vi "cDAQ Abort Digitize.vi"(8 "error in":errorcluster, 11 "cdaq session in":T1={"mclk [Hz]"=12800000.0, "ADC task"="", "mclk reference"="", "fs [Hz]"=50000.0, "queue adc cmd"=refnum, "queue adc data"=refnum, "adc proc ref"=refnum, "channels"=[], "last channels"=[], "timeout"=timestamp(0 s since 1904-01-01), "N"=1000, "mclk mode"=enum."Free running", "ext mclk source"=""} {"last channels"."Channel id" min=0 step=1; "channels"."Channel id" min=0 step=1}) -> (0 "error out":errorcluster, 3 "cdaq session out":T1={"mclk [Hz]"=12800000.0, "ADC task"="", "mclk reference"="", "fs [Hz]"=50000.0, "queue adc cmd"=refnum, "queue adc data"=refnum, "adc proc ref"=refnum, "channels"=[], "last channels"=[], "timeout"=timestamp(0 s since 1904-01-01), "N"=1000, "mclk mode"=enum."Free running", "ext mclk source"=""} {"last channels"."Channel id" min=0 step=1; "channels"."Channel id" min=0 step=1})   [LabVIEW 2020]
uses:
  cDAQ Session.ctl
  low_level_old/cdaq_anal_adc_command.ctl
  low_level_old/cdaq_anal_adc_data.ctl
  cDAQ Virtual Channel.ctl
  cDAQ Master Clock Mode.ctl
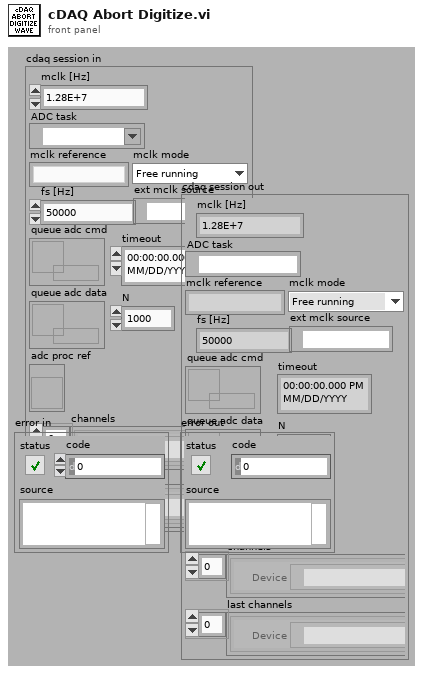
[diagram p1: front panel]
types:
  T1 = typedef "cDAQ Session.ctl" = cluster{"mclk [Hz]":dbl, "ADC task":refnum<k21>, "mclk reference":string, "fs [Hz]":dbl, "queue adc cmd":refnum<queue>, "queue adc data":refnum<queue>, "adc proc ref":refnum<vi>, "channels":T2[], "last channels":T2[], "timeout":timestamp, "N":i32, "mclk mode":T3, "ext mclk source":tag}
  T2 = typedef "cDAQ Virtual Channel.ctl" = cluster{"Device":tag, "Channel id":i32, "btn clr":bool, "btn up":bool, "btn down":bool}
  T3 = typedef "cDAQ Master Clock Mode.ctl" = enum16{"Free running", "Export master clock", "Import master clock"}
  T4 = typedef "cdaq_anal_adc_command.ctl" = cluster{"sample to get":i32, "stop":bool, "abort":bool}
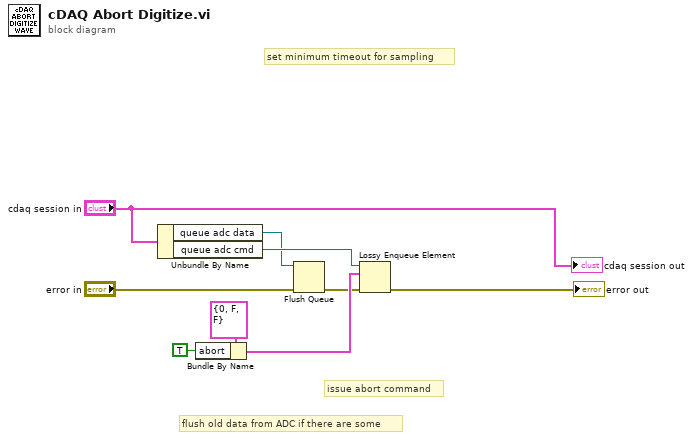
[diagram p0: block diagram]
diagram:
  # "set minimum timeout for sampling"
  # "issue abort command"
  # "flush old data from ADC if there are some"
  n1 = Unbundle By Name("cdaq session in") -> ("queue adc data"=w4:refnum<queue>, "queue adc cmd"=w8:refnum<queue>)
  n2 = Bundle By Name(cluster=T4 {"sample to get"=0, "stop"=FALSE, "abort"=FALSE} ("adc cmd"), "abort"=TRUE) -> (w7:T4)
  n3 = Flush Queue(queue=w4, error in (no error)="error in") -> (error out=w6:errorcluster)  [unwired: 2 out]
  n4 = Lossy Enqueue Element(queue=w8, element=w7, error in (no error)=w6) -> (error out=→"error out":errorcluster)  [unwired: 3 out]
  "cdaq session out" <- "cdaq session in"
